vi "Write FP Control.vi"(6 "Field name":string, 8 "error in (no error)":errorcluster, 9 "Control Value":variant, 10 "Control Name":string="Configuration", 11 "Measure Object in":refnum<class "Template Module.lvclass">) -> (0 "error out":errorcluster, 3 "Measure Object out":refnum<class "Template Module.lvclass">)   [LabVIEW 2019, in "Template Module.lvclass"]
uses:
  Template Module.lvclass
  Template Module.lvclass/Template Module.ctl
  Read Front Panel ref.vi
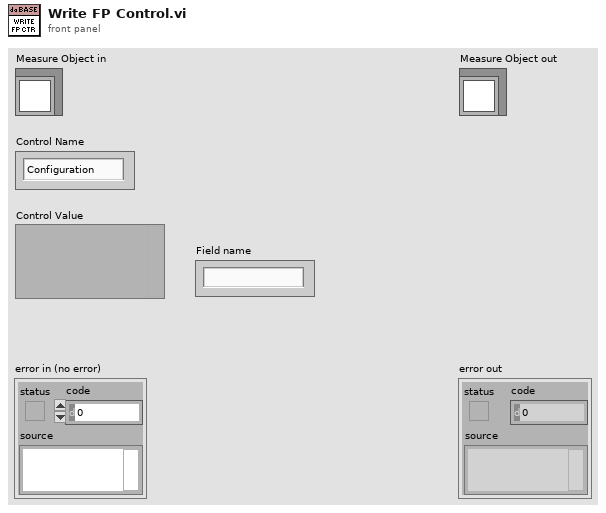
[diagram p1: front panel]
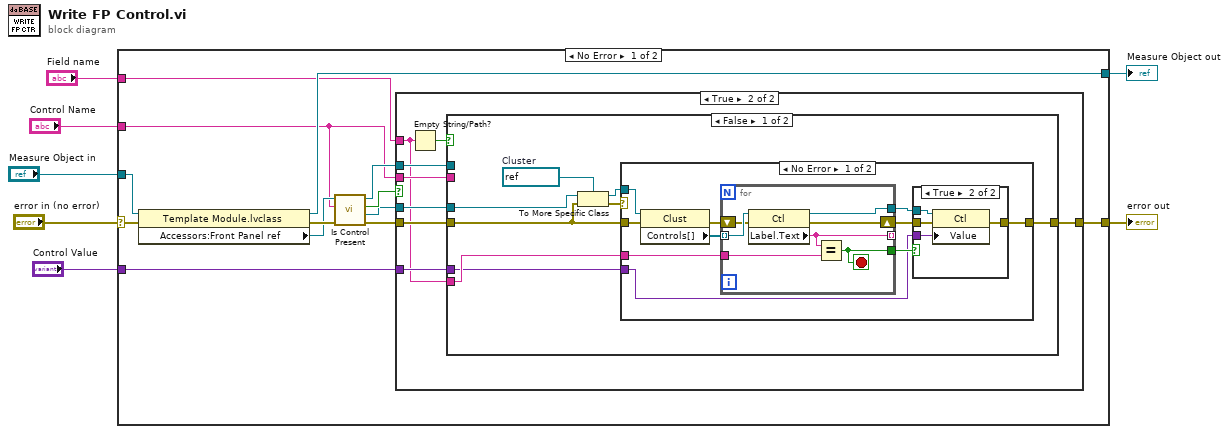
[diagram p0: block diagram]
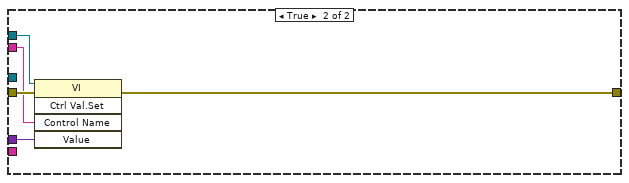
[diagram p5: hidden frame]
diagram:
  n1 = case shown="No Error" "error in (no error)" {
    selector: "error in (no error)" -> [w20 w67]
    tunnel: [w17 w67] -> w6
    tunnel: [w18 w66] -> w4
    tunnel: "Measure Object in" -> [w19 w66]
    tunnel: "Control Name" -> [w11 _]
    tunnel: "Control Value" -> [w10 _]
    tunnel: "Field name" -> [w9 _]
    frame No Error {
      n2 = property class="Template Module.lvclass"(reference=w19, error in=w20) -> (reference out=w18:refnum<class "Template Module.lvclass">, error out=w16:errorcluster, "Accessors:Front Panel ref"=w14:refnum<vi>)
      n3 = call "Is Control Present.vi"("Error In"=w16, "Control label"=w11, "VI ref"=w14) -> ("Error Out"=w15:errorcluster, "Ctl Refnum"=w8:refnum<vi>, "Present"=w12:bool, "VI ref out"=w13:refnum<vi>)  [unwired: 5 in]
      n4 = case shown="True" w12 {
        tunnel: [w21 w29] -> w17
        tunnel: w15 -> [w21 w28]
        tunnel: w13 -> [_ w27]
        tunnel: w11 -> [_ w26]
        tunnel: w10 -> [_ w25]
        tunnel: w9 -> [_ w22]
        tunnel: w8 -> [_ w23]
        frame False {
        }
        frame True {
          n5 = Empty String/Path?(string/path=w22) -> (empty?=w24:bool)
          n6 = case shown="False" w24 {
            tunnel: [w30 w65] -> w29
            tunnel: w28 -> [w33 w64]
            tunnel: w27 -> [_ w63]
            tunnel: w26 -> [_ w62]
            tunnel: w25 -> [w31 w61]
            tunnel: w23 -> [w37 _]
            tunnel: w22 -> [w32 _]
            frame False {
              w36 = refnum<vi> refnum  # Cluster
              n7 = To More Specific Class(target class=w36, reference=w37, error in=w33) -> (specific class reference=w34:refnum<vi>, error out=w35:errorcluster)
              n8 = case shown="No Error" w35 {
                tunnel: w34 -> [w46 _]
                tunnel: w33 -> [w45 w60]
                tunnel: w32 -> [w43 _]
                tunnel: w31 -> [w40 _]
                tunnel: [w38 w60] -> w30
                frame No Error {
                  n9 = property class="Clust"(reference=w46, error in=w45) -> (error out=w44:errorcluster, "Controls[]"=w47:refnum<vi>[])  [unwired: 1 out]
                  n10 = for {
                    tunnel: w47 -> [w59] mode=indexing
                    tunnel: [w56] -> _ mode=indexing
                    shift-right: [w57] -> w39
                    shift-left: w44 -> [w58]
                    tunnel: w43 -> [w55]
                    tunnel: [w54] -> w41
                    tunnel: [w53] -> w42
                    stop <- w53 stop-if-true
                    n11 = property class="Ctl"(reference=w59, error in=w58) -> (reference out=w54:refnum<vi>, error out=w57:errorcluster, "Label.Text"=w56:string)
                    n12 = Equal?(x=w56, y=w55) -> (x = y?=w53:bool)
                  }
                  n13 = case shown="True" w42 {
                    tunnel: w41 -> [_ w52]
                    tunnel: w40 -> [_ w51]
                    tunnel: w39 -> [w48 w50]
                    tunnel: [w48 w49] -> w38
                    frame False {
                    }
                    frame True {
                      n14 = property class="Ctl"(reference=w52, error in=w50, "Value"=w51) -> (error out=w49:errorcluster)  [unwired: 1 out]
                    }
                  }
                }
                frame Error {
                }
              }
            }
            frame True {
              n15 = invoke class="VI" method="Ctrl Val.Set"(reference=w63, error in=w64, "Control Name"=w62, "Value"=w61) -> (error out=w65:errorcluster)  [unwired: 1 in, 4 out]
            }
          }
        }
      }
    }
    frame Error {
    }
  }
  "error out" <- w6
  "Measure Object out" <- w4
